vi "test_libssh2_userauth_publickey_frommemory.vi"() -> ()   [LabVIEW 2017, in "integration_tests.lvlib"]
uses:
  integration_tests.lvlib
  libssh2/libssh2_session_handshake_tcp.vi
  libssh2/libssh2_init_default.vi
  libssh2/libssh2_session_init_ex.vi
  <vilib>/Utility/tcp.llb/TCP Get Raw Net Object.vi
  libssh2/libssh2_session_handshake_socket.vi
  libssh2/libssh2.lvlib
  support/support.lvlib
  <vilib>/PNR/Transparent Assertions/Transparent Assertions/Transparent Assertions.lvlib
panel:
  out "error out":errorcluster
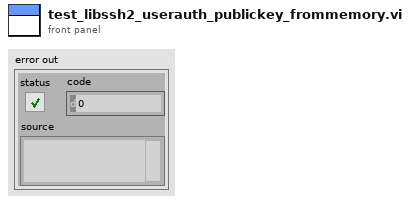
[diagram p1: front panel]
types:
  T1 = typedef "libssh2.lvlib/Session Refnum.ctl" = refnum<k1>
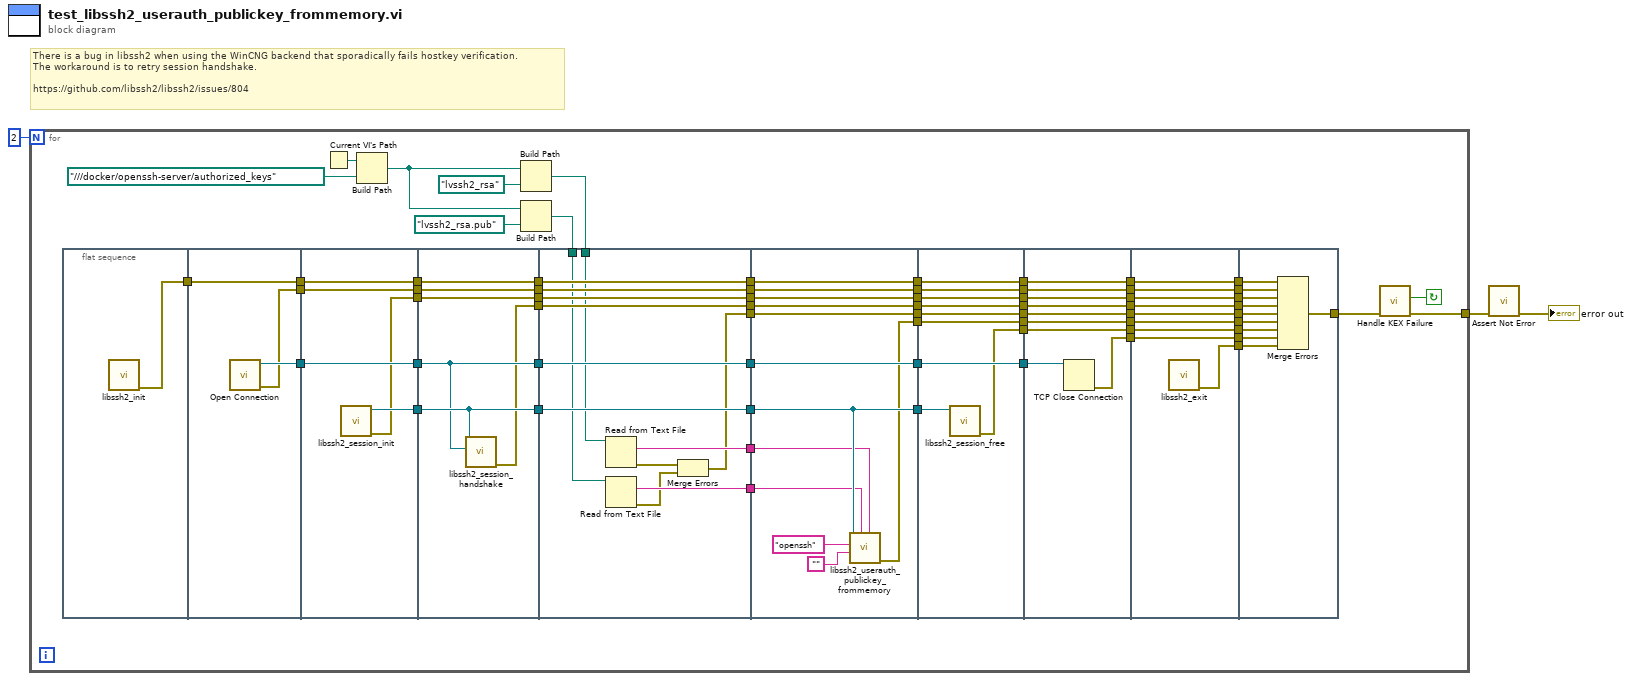
[diagram p0: block diagram]
diagram:
  # "There is a bug in libssh2 when using the WinCNG backend that sporadically fails hostkey verification.\nThe workaround is to retry session handshake.\n\nhttps://github.com/libssh2/libssh2/issues/804"
  n1 = for {
    N: 2 -> [_]
    tunnel: [w8] -> w2
    stop <- w9 continue-if-true
    n2 = flat-sequence {
      tunnel: [w71] -> w70
      tunnel: [w74] -> w69
      tunnel: w70 -> [w73]
      tunnel: [w73] -> w68
      tunnel: [w72] -> w67
      tunnel: w69 -> [w79]
      tunnel: [w79] -> w66
      tunnel: w68 -> [w78]
      tunnel: [w78] -> w65
      tunnel: w67 -> [w77]
      tunnel: [w77] -> w64
      tunnel: [w76] -> w63
      tunnel: [w75] -> w62
      tunnel: w66 -> [w81]
      tunnel: [w81] -> w61
      tunnel: w65 -> [w85]
      tunnel: [w85] -> w60
      tunnel: w64 -> [w84]
      tunnel: [w84] -> w59
      tunnel: [w83] -> w58
      tunnel: w63 -> [w83]
      tunnel: w62 -> [w82]
      tunnel: [w82] -> w57
      tunnel: [w80] -> w56
      tunnel: w61 -> [w98]
      tunnel: [w98] -> w55
      tunnel: w60 -> [w97]
      tunnel: [w97] -> w54
      tunnel: w59 -> [w96]
      tunnel: [w96] -> w53
      tunnel: w58 -> [w95]
      tunnel: [w95] -> w52
      tunnel: w57 -> [w94]
      tunnel: [w94] -> w51
      tunnel: w56 -> [w93]
      tunnel: [w93] -> w50
      tunnel: [w92] -> w49
      tunnel: [w91] -> w48
      tunnel: w12 -> [w90]
      tunnel: w11 -> [w89]
      tunnel: [w86] -> w47
      tunnel: w55 -> [w110]
      tunnel: [w110] -> w46
      tunnel: w54 -> [w109]
      tunnel: [w109] -> w45
      tunnel: w53 -> [w108]
      tunnel: [w108] -> w44
      tunnel: w52 -> [w105]
      tunnel: w51 -> [w107]
      tunnel: [w107] -> w43
      tunnel: w50 -> [w106]
      tunnel: [w106] -> w42
      tunnel: [w105] -> w41
      tunnel: w49 -> [w102]
      tunnel: w48 -> [w101]
      tunnel: w47 -> [w100]
      tunnel: [w100] -> w40
      tunnel: [w99] -> w7
      tunnel: w46 -> [w119]
      tunnel: [w119] -> w39
      tunnel: w45 -> [w118]
      tunnel: [w118] -> w38
      tunnel: w44 -> [w117]
      tunnel: [w117] -> w37
      tunnel: w43 -> [w116]
      tunnel: [w116] -> w36
      tunnel: w42 -> [w115]
      tunnel: [w115] -> w35
      tunnel: [w114] -> w34
      tunnel: w41 -> [w113]
      tunnel: w40 -> [w112]
      tunnel: [w112] -> w33
      tunnel: w7 -> [w111]
      tunnel: [w111] -> w6
      tunnel: w39 -> [w128]
      tunnel: w38 -> [w127]
      tunnel: [w127] -> w32
      tunnel: w37 -> [w126]
      tunnel: [w126] -> w31
      tunnel: [w125] -> w30
      tunnel: w36 -> [w124]
      tunnel: [w124] -> w29
      tunnel: w35 -> [w123]
      tunnel: [w123] -> w28
      tunnel: [w122] -> w27
      tunnel: w34 -> [w122]
      tunnel: w33 -> [w121]
      tunnel: [w121] -> w26
      tunnel: w6 -> [w120]
      tunnel: [w120] -> w5
      tunnel: w32 -> [w137]
      tunnel: [w137] -> w25
      tunnel: w31 -> [w136]
      tunnel: [w136] -> w24
      tunnel: w30 -> [w135]
      tunnel: [w135] -> w23
      tunnel: [w134] -> w22
      tunnel: w29 -> [w133]
      tunnel: [w133] -> w21
      tunnel: w28 -> [w132]
      tunnel: [w132] -> w20
      tunnel: [w131] -> w19
      tunnel: w27 -> [w131]
      tunnel: w26 -> [w130]
      tunnel: [w130] -> w18
      tunnel: w5 -> [w129]
      tunnel: [w129] -> w4
      tunnel: w25 -> [w147]
      tunnel: w24 -> [w146]
      tunnel: w23 -> [w145]
      tunnel: w22 -> [w144]
      tunnel: w21 -> [w143]
      tunnel: w20 -> [w142]
      tunnel: w19 -> [w141]
      tunnel: w18 -> [w140]
      tunnel: [w139] -> w10
      tunnel: w4 -> [w138]
      frame #0 {
        n3 = call-poly "libssh2_init.vi"() -> ("error out"=w71:errorcluster)  [unwired: 11 in]
      }
      frame #1 {
        n4 = call "Open Connection.vi"() -> ("error out"=w72:errorcluster, "connection ID"=w74:refnum<k5>)  [unwired: 10 in]
      }
      frame #2 {
        n5 = call "libssh2_session_init.vi"() -> ("error out"=w75:errorcluster, "session"=w76:T1)  [unwired: 10 in]
      }
      frame #3 {
        n6 = call-poly "libssh2_session_handshake.vi"("tcp connection"=w81, "session"=w83) -> ("error out"=w80:errorcluster)  [unwired: 9 in]
      }
      frame #4 {
        n7 = Read from Text File(file (use dialog)=w90) -> (text=w91:string, error out=w87:errorcluster)  [unwired: 3 in, 2 out]
        n8 = Read from Text File(file (use dialog)=w89) -> (text=w92:string, error out=w88:errorcluster)  [unwired: 3 in, 2 out]
        n9 = Merge Errors(w87, w88) -> (w86:errorcluster)
      }
      frame #5 {
        n10 = call "libssh2_userauth_publickey_frommemory.vi"("private key data"=w101, "public key data"=w102, "passphrase"="", "username"="openssh", "session"=w105) -> ("error out"=w99:errorcluster)  [unwired: 6 in]
      }
      frame #6 {
        n11 = call "libssh2_session_free.vi"("session"=w113) -> ("error out"=w114:errorcluster)  [unwired: 10 in]
      }
      frame #7 {
        n12 = TCP Close Connection(connection ID=w128) -> (error out=w125:errorcluster)  [unwired: 2 in, 1 out]
      }
      frame #8 {
        n13 = call "libssh2_exit.vi"() -> ("error out"=w134:errorcluster)  [unwired: 11 in]
      }
      frame #9 {
        n14 = Merge Errors(w147, w146, w143, w142, w140, w138, w141, w145, w144) -> (w139:errorcluster)
      }
    }
    n15 = Current VI's Path() -> (path=w13:path)
    n16 = Build Path(base path=w13, name or relative path=path "../../../docker/openssh-server/authorized_keys" ("stripped path")) -> (appended path=w14:path)
    n17 = Build Path(base path=w14, name or relative path=path "lvssh2_rsa" ("stripped path")) -> (appended path=w12:path)
    n18 = Build Path(base path=w14, name or relative path=path "lvssh2_rsa.pub" ("stripped path")) -> (appended path=w11:path)
    n19 = call "Handle KEX Failure.vi"("error in (no error)"=w10) -> ("error out"=w8:errorcluster, "KEX Failure"=w9:bool)  [unwired: 9 in]
  }
  n20 = call <vilib>:"Assert Not Error.vi"("error in (no error)"=w2) -> ("error out"=→"error out":errorcluster)  [unwired: 10 in]
